vi "test_1_直接调用DLL内的函数.vi"   [LabVIEW 2012]
uses:
  LabView4Las.dll
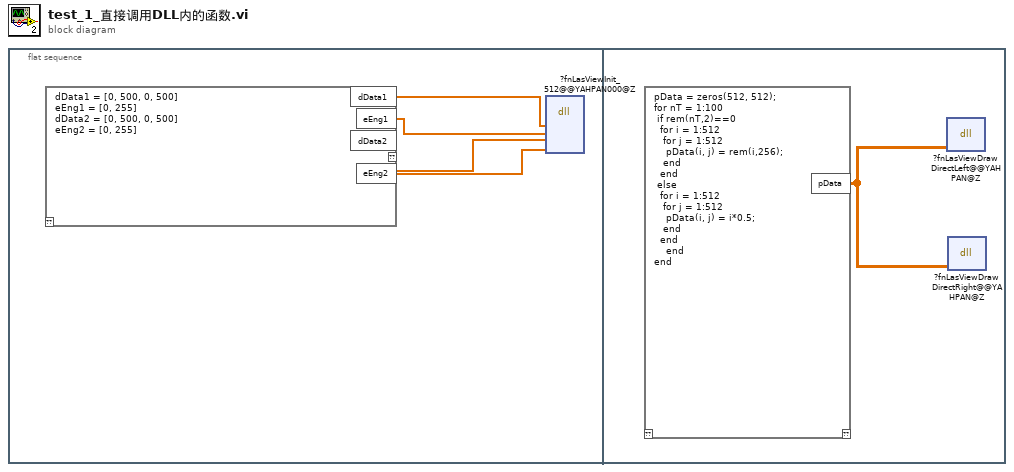
[diagram p0: block diagram]
diagram:
  n1 = flat-sequence {
    frame #0 {
      n2 = script code="dData1 = [0, 500, 0, 500]\neEng1 = [0, 255]\ndData2 = [0, 500, 0, 500]\neEng2 = [0, 255]"() -> ("dData1"=w4:cdb[], "eEng1"=w3:cdb[], "dData2"=w2:cdb[], "eEng2"=w1:cdb[])  [unwired: 1 in, 1 out]
      n3 = dll-call lib="C:/Developer/labview/dll2/LabView4Las.dll" fn="?fnLasViewInit_512@@YAHPAN000@Z"("dData1"=w4, "eEng1"=w3, "dData2"=w2, "eEng2"=w1) -> ()  [unwired: 8 in, 2 out]
    }
    frame #1 {
      n4 = script code="pData = zeros(512, 512);\nfor nT = 1:100\n\tif rem(nT,2)==0\n\t\tfor i = 1:512\n\t\t\tfor j = 1:512\n\t\t\t\tpData(i, j) = rem(i,256);\n\t\t\tend\n\t\tend\n\telse\n\t\tfor i = 1:512\n\t\t\tfor j = 1:512\n\t\t\t\tpData(i, j) = i*0.5;\n\t\t\tend\n\t\tend\n    end\nend"() -> ("pData"=w5:cdb[][])  [unwired: 1 in, 1 out]
      n5 = dll-call lib="C:/Developer/labview/dll2/LabView4Las.dll" fn="?fnLasViewDrawDirectLeft@@YAHPAN@Z"("pData"=w5) -> ()  [unwired: 5 in, 2 out]
      n6 = dll-call lib="C:/Developer/labview/dll2/LabView4Las.dll" fn="?fnLasViewDrawDirectRight@@YAHPAN@Z"("pData"=w5) -> ()  [unwired: 5 in, 2 out]
    }
  }
